vi "SetSettings.vi"(8 "error in (no error)":errorcluster, 10 "Variant":variant, 11 "ChromaAcLoad in":refnum<class "ChromaAcLoad.lvclass">) -> (0 "error out":errorcluster, 3 "ChromaAcLoad Out":refnum<class "ChromaAcLoad.lvclass">)   [LabVIEW 2018, in "AcPwrPlugins.lvlib" / "ChromaAcLoad.lvclass"]
doc: "This VI retrieves a boolean status to see if the instrument can conduct measurements while the device is changing modes or turning off and on."
uses:
  ChromaAcLoad.lvclass
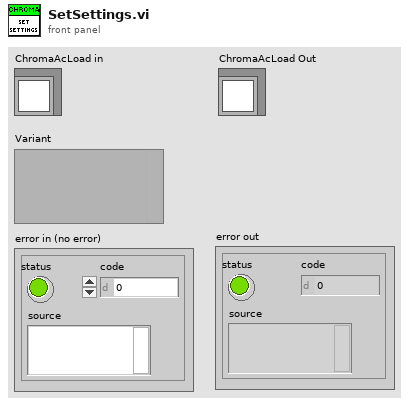
[diagram p1: front panel]
types:
  T1 = typedef "AcPwrPlugins.lvlib/ChromaAcLoad.lvclass/Device(s)Settings.ctl" = cluster{"Configuration Mode":enum16{"Constant Voltage (DC)", "Constant Power (DC)", "Constant Power (AC)", "Constant Current (DC)", "Constant Current (AC)", "Constant Resistance (DC)", "Constant Resistance (AC)", "Rectified Mode (DC)", "Inrush (AC)", "RLC CP (AC)", "RLC (AC)"}, "Phases":cluster{"Handle":string, "Name":string, "Phase Select":i32, "Instrument Options":string, "id query (T)":bool, "reset device (T)":bool, "Load Short Circuited":bool, "Line Synchronization":bool, "Load Current (A/Arms)":dbl, "Load Voltage (V/Vrms)":dbl, "Load Power (W)":dbl, "Load Resistance (Ohms)":dbl, "Load Current Peak Limit (A)":dbl, "Load Current Limit (A/Arms)":dbl, "Load Power Limit (W)":dbl, "Synch Frequency (Hz)":dbl, "Priority":enum16{"CF Only", "PF Only", "Both (CF)", "Both (PF)"}, "Crest Factor":dbl, "Power Factor":dbl, "Slew Rate":cluster{"Rise Slew Rate (A/ms)":i32, "Fall Slew Rate (A/ms)":i32}, "LC/RLC Mode":cluster{"Capacitance (uF)":i32, "Inductance (uH)":i32, "Series Resistance (Ohm)":dbl, "Parallel Resistance (Ohm)":dbl}, "Timing":cluster{"TimingOn":enum16{""}, "Hours":u32, "Minutes":u32, "Seconds":dbl, "CutoffVoltage":dbl}, "Connected":bool}[], "MeasName":string}
  T2 = typedef "AcPwrPlugins.lvlib/ChromaAcLoad.lvclass/Measurements.ctl" = cluster{"Handle":string, "Name":string, "Enabled":bool, "Measurement Value":dbl, "Hold Peak Current Measurement":bool, "btnMeasFetch":bool, "ProtectionStatusString":string, "Measurement Type":T3}[]
  T3 = typedef "AcPwrPlugins.lvlib/ChromaAcLoad.lvclass/MeasurementType.ctl" = enum16{"Voltage (Vrms or V)", "Current (Arms or A)", "Power (W)", "Peak Voltage (V)", "Peak Current (A)", "Peak Power (W)", "Frequency (Hz)", "Resistance (Ohms)", "Voltage Overshoot (V)", "Positive Peak Current (A)", "Voltage Undershoot (V)", "Negative Peak Current (A)", "Apparent Power (VA)", "Reacitive Power (VAR)", "Voltage THD", "Power Factor", "Current's Crest Factor"}
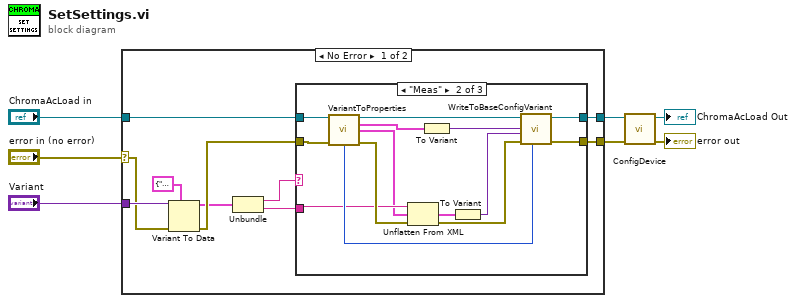
[diagram p0: block diagram]
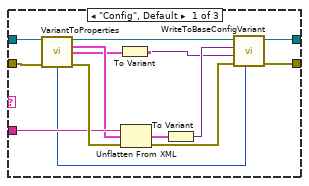
[diagram p2: hidden frame]
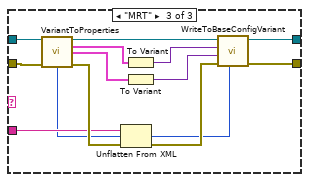
[diagram p3: hidden frame]
diagram:
  n1 = case shown="No Error" "error in (no error)" {
    selector: "error in (no error)" -> [w13 w61]
    tunnel: [w16 w61] -> w4
    tunnel: "ChromaAcLoad in" -> [w17 w60]
    tunnel: "Variant" -> [w14 _]
    tunnel: [w15 w60] -> w2
    frame No Error {
      n2 = Variant To Data(error in=w13, type=cluster{string, string} {"", ""}, Variant=w14) -> (data=w10:cluster{string, string}, error out=w11:errorcluster)
      n3 = Unbundle(w10) -> (w8:string, w9:string)
      n4 = case shown="\"Meas\"" w8 {
        tunnel: [w24 w40 w54] -> w16
        tunnel: w17 -> [w26 w42 w56]
        tunnel: [w21 w38 w51] -> w15
        tunnel: w11 -> [w31 w45 w59]
        tunnel: w9 -> [w29 w36 w57]
        frame "Config", Default {
          n5 = call "VariantToProperties.vi"("ChromaAcLoad"=w26, "error in (no error)"=w31) -> ("ChromaAcLoad"=w22:refnum<class "ChromaAcLoad.lvclass">, "Device Properties"=w27:T1, "Meas"=w20:T2, "Measurement Refresh Time (ms)"=w18:u32, "error out"=w30:errorcluster)  [unwired: 7 in, 2 out]
          n6 = To Variant(anything=w20) -> (Variant=w19:variant)
          n7 = Unflatten From XML(xml string=w29, type=w27, error in (no error)=w30) -> (value=w28:T1, error out=w25:errorcluster)
          n8 = To Variant(anything=w28) -> (Variant=w23:variant)
          n9 = call "WriteToBaseConfigVariant.vi"("Measurement Refresh Time (ms)"=w18, "error in (no error)"=w25, "Meas"=w19, "Config"=w23, "ChromaAcLoad in"=w22) -> ("error out"=w24:errorcluster, "ChromaAcLoad out"=w21:refnum<class "ChromaAcLoad.lvclass">)  [unwired: 5 in]
        }
        frame "Meas" {
          n10 = call "VariantToProperties.vi"("ChromaAcLoad"=w42, "error in (no error)"=w45) -> ("ChromaAcLoad"=w39:refnum<class "ChromaAcLoad.lvclass">, "Device Properties"=w33:T1, "Meas"=w35:T2, "Measurement Refresh Time (ms)"=w37:u32, "error out"=w44:errorcluster)  [unwired: 7 in, 2 out]
          n11 = Unflatten From XML(xml string=w36, type=w35, error in (no error)=w44) -> (value=w43:T2, error out=w41:errorcluster)
          n12 = To Variant(anything=w33) -> (Variant=w32:variant)
          n13 = To Variant(anything=w43) -> (Variant=w34:variant)
          n14 = call "WriteToBaseConfigVariant.vi"("Measurement Refresh Time (ms)"=w37, "error in (no error)"=w41, "Meas"=w34, "Config"=w32, "ChromaAcLoad in"=w39) -> ("error out"=w40:errorcluster, "ChromaAcLoad out"=w38:refnum<class "ChromaAcLoad.lvclass">)  [unwired: 5 in]
        }
        frame "MRT" {
          n15 = call "VariantToProperties.vi"("ChromaAcLoad"=w56, "error in (no error)"=w59) -> ("ChromaAcLoad"=w52:refnum<class "ChromaAcLoad.lvclass">, "Device Properties"=w47:T1, "Meas"=w50:T2, "Measurement Refresh Time (ms)"=w48:u32, "error out"=w58:errorcluster)  [unwired: 7 in, 2 out]
          n16 = Unflatten From XML(xml string=w57, type=w48, error in (no error)=w58) -> (value=w46:u32, error out=w55:errorcluster)
          n17 = To Variant(anything=w47) -> (Variant=w53:variant)
          n18 = To Variant(anything=w50) -> (Variant=w49:variant)
          n19 = call "WriteToBaseConfigVariant.vi"("Measurement Refresh Time (ms)"=w46, "error in (no error)"=w55, "Meas"=w49, "Config"=w53, "ChromaAcLoad in"=w52) -> ("error out"=w54:errorcluster, "ChromaAcLoad out"=w51:refnum<class "ChromaAcLoad.lvclass">)  [unwired: 5 in]
        }
      }
    }
    frame Error {
    }
  }
  n20 = call-dynamic "ConfigDevice.vi"("error in (no error)"=w4, "ChromaAcLoad in"=w2) -> ("error out"=→"error out":errorcluster, "ChromaAcLoad out"=→"ChromaAcLoad Out":refnum<class "ChromaAcLoad.lvclass">)  [unwired: 8 in]
